vi "PhotonPipelineResult_GetTargets.vi"(11 "PhotonPipelineResult_REF":T7) -> (3 "Targets":T1[](array[typedef]) {"AltCameraToTarget"."TRANSLATION3D"."Z" format="%14.3f"; "AltCameraToTarget"."TRANSLATION3D"."Y" format="%14.3f"; "AltCameraToTarget"."TRANSLATION3D"."X" format="%14.3f"; "BestCameraToTarget"."TRANSLATION3D"."Z" format="%14.3f"; "BestCameraToTarget"."TRANSLATION3D"."Y" format="%14.3f"; "BestCameraToTarget"."TRANSLATION3D"."X" format="%14.3f"})   [LabVIEW 2019, in "PhotonVisionLib.lvlib"]
doc: "Returns the targets in this pipeline result. If there are no targets, this method will return an empty target array. \n\nInputs:\n - PipelineResult -- Parsed PipelineResult cluster.\n\nOutputs:\n - Targets -- Array of Target clusters."
uses:
  PhotonVisionLib.lvlib
  TypeDef/PhotonPipelineResultType.ctl
  TypeDef/PhotonTrackedTargetType.ctl
  TypeDef/TargetCornerType.ctl
  <vilib>/Rock Robotics/WPI/ThirdParty/JAS_Junk/TrajLib/TypeDef/TRANSFORM3D.ctl
  <vilib>/Rock Robotics/WPI/ThirdParty/JAS_Junk/TrajLib/TypeDef/TRANSLATION3D.ctl
  <vilib>/Rock Robotics/WPI/ThirdParty/JAS_Junk/TrajLib/TypeDef/ROTATION3D.ctl
  <vilib>/Rock Robotics/WPI/ThirdParty/JAS_Junk/TrajLib/TypeDef/QUATERNION.ctl
  TypeDef/PhotonMultiTargetPNPResultType.ctl
  TypeDef/PhotonPNPResultType.ctl
  <vilib>/Rock Robotics/WPI/ThirdParty/JAS_Junk/TrajLib/Trajectory_Library.lvlib
  Ref/PhotonPipelineResult_REF.ctl
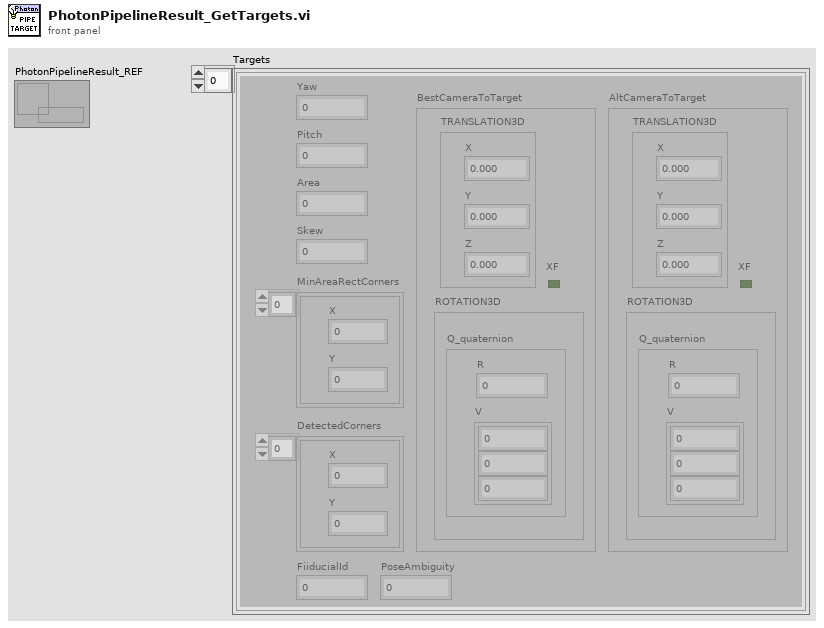
[diagram p1: front panel]
types:
  T1 = typedef "PhotonVisionLib.lvlib/PhotonTrackedTargetType.ctl" = cluster{"Yaw":dbl, "Pitch":dbl, "Area":dbl, "Skew":dbl, "MinAreaRectCorners":T2[], "BestCameraToTarget":T3, "FiiducialId":i32, "AltCameraToTarget":T3, "PoseAmbiguity":dbl, "DetectedCorners":T2[]}
  T2 = typedef "PhotonVisionLib.lvlib/TargetCornerType.ctl" = cluster{"X":dbl, "Y":dbl}
  T3 = typedef "Trajectory_Library.lvlib/TRANSFORM3D.ctl" = cluster{"TRANSLATION3D":T4, "ROTATION3D":T5, "XF":bool}
  T4 = typedef "Trajectory_Library.lvlib/TRANSLATION3D.ctl" = cluster{"X":dbl, "Y":dbl, "Z":dbl}
  T5 = typedef "Trajectory_Library.lvlib/ROTATION3D.ctl" = cluster{"Q_quaternion":T6}
  T6 = typedef "Trajectory_Library.lvlib/QUATERNION.ctl" = cluster{"R":dbl, "V":dbl[]}
  T7 = typedef "PhotonVisionLib.lvlib/PhotonPipelineResult_REF.ctl" = refnum<data-value>
  T8 = typedef "PhotonVisionLib.lvlib/PhotonPipelineResultType.ctl" = cluster{"TargetCount":i32, "Latency_MilliSec":dbl, "Targets":T1[], "TimeStampSec":dbl, "PhotonMultiTargetPNPResult":T9}
  T9 = typedef "PhotonVisionLib.lvlib/PhotonMultiTargetPNPResultType.ctl" = cluster{"PhotonPNPResult":T10, "FiducialIDsUsed":i16[]}
  T10 = typedef "PhotonVisionLib.lvlib/PhotonPNPResultType.ctl" = cluster{"IsPresent":bool, "bestReprojErr":dbl, "altReprojErr":dbl, "ambiguity":dbl, "Best":T3, "Alt":T3}
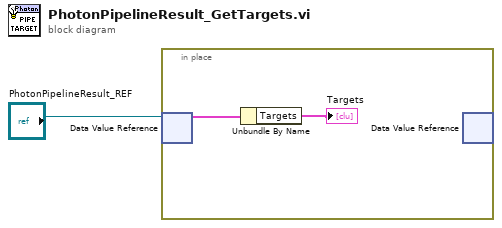
[diagram p0: block diagram]
diagram:
  n1 = in-place {
    n2 = in-place-dvr #1("PhotonPipelineResult_REF") -> (w3:T8)  [unwired: 1 out]
    n3 = Unbundle By Name(w3) -> ("Targets"=→"Targets":T1[])
    n4 = in-place-dvr #1() -> ()  [unwired: 1 in, 2 out]
  }
